vi "niP2P Property Node.vi"   [LabVIEW 2010]
doc: "This Property Node is configured to access peer-to-peer stream properties."
uses:
  resource/objmgr/PeerToPeerStream.rc
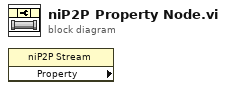
[diagram p0: block diagram]
diagram:
  n1 = property class="niP2P Stream" props=[]() -> ()  [unwired: 2 in, 3 out]
